vi "Dequeue Master and Local.vi"(8 "error in (no error)":errorcluster, 10 "Master Queue In":refnum<queue>, 11 "UI In":refnum<queue>) -> (0 "error out":errorcluster, 1 "Message Data":variant, 2 "Message":string, 3 "UI Out":refnum<queue>)   [LabVIEW 2013, in "Cal Inst.lvlib" / "Cal Inst Message Queue.lvlib"]
uses:
  Cal Inst Message Queue.lvlib
  Message Cluster.ctl
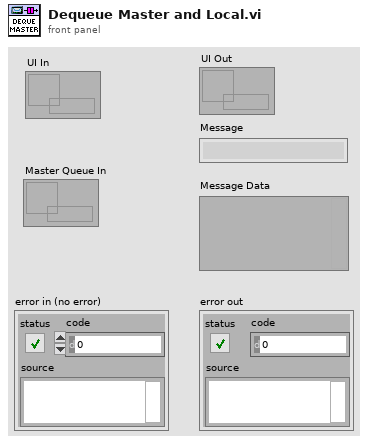
[diagram p1: front panel]
types:
  T1 = typedef "Cal Inst.lvlib/Cal Inst Message Queue.lvlib/Message Cluster.ctl" = cluster{"Message":string, "Message Data":variant}
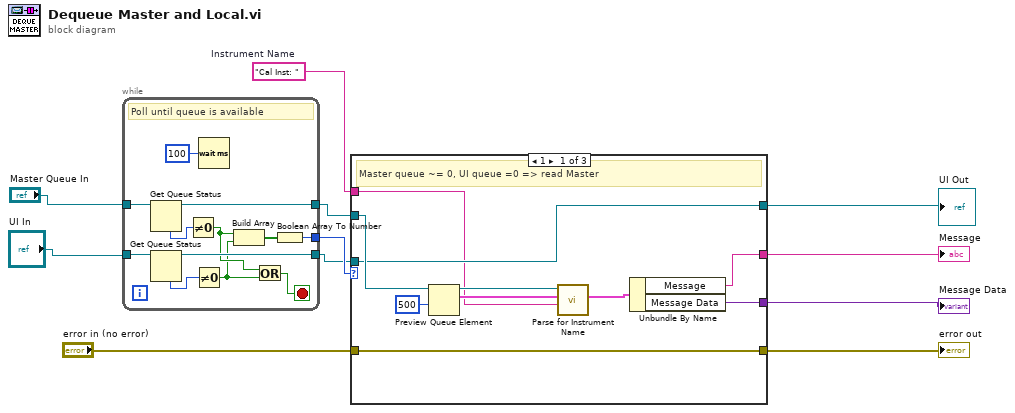
[diagram p0: block diagram]
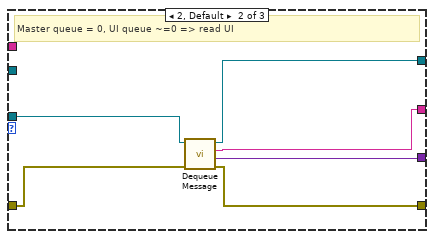
[diagram p2: hidden frame]
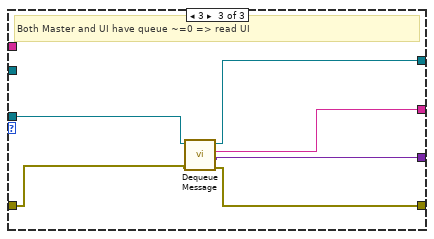
[diagram p3: hidden frame]
diagram:
  w6 = "Cal Inst: "  # Instrument Name
  n1 = while {
    tunnel: "UI In" -> [w23]
    tunnel: "Master Queue In" -> [w20]
    tunnel: [w18] -> w11
    tunnel: [w17] -> w10
    tunnel: [w16] -> w9
    stop <- w14 stop-if-true
    # "Poll until queue is available"
    n2 = Get Queue Status(queue=w20) -> (queue out=w17:refnum<queue>, # elements in queue=w21:i32)  [unwired: 2 in, 6 out]
    n3 = Get Queue Status(queue=w23) -> (queue out=w16:refnum<queue>, # elements in queue=w22:i32)  [unwired: 2 in, 6 out]
    n4 = Not Equal To 0?(x=w21) -> (x != 0?=w13:bool)
    n5 = Not Equal To 0?(x=w22) -> (x != 0?=w12:bool)
    n6 = Wait (ms)(milliseconds to wait=u32 100) -> ()  [unwired: 1 out]
    n7 = Build Array(w13, w12) -> (w19:bool[])
    n8 = Or(x=w13, y=w12) -> (x .or. y?=w14:bool)
    n9 = Boolean Array To Number(Boolean array=w19) -> (number=w18:u32)
  }
  n10 = case shown="1" w11 {
    tunnel: w10 -> [w30 _ _]
    tunnel: w9 -> [w26 w39 w40]
    tunnel: "error in (no error)" -> [w31 w38 w45]
    tunnel: [w26 w34 w41] -> w3
    tunnel: [w33 w35 w42] -> w2
    tunnel: [w32 w36 w43] -> w1
    tunnel: [w31 w37 w44] -> w7
    tunnel: w6 -> [w25 _ _]
    frame 1 {
      # "Master queue ~= 0, UI queue =0 => read Master"
      n11 = Preview Queue Element(queue=w30, timeout in ms (-1)=500) -> (queue out=w29:refnum<queue>, element=w28:T1)  [unwired: 1 in, 2 out]
      n12 = call "Parse for Instrument Name.vi"("Instrument Name"=w25, "Message In"=w28, "Message Queue"=w29) -> ("Message Out"=w27:T1)  [unwired: 8 in]
      n13 = Unbundle By Name(w27) -> ("Message"=w33:string, "Message Data"=w32:variant)
    }
    frame 2, Default {
      # "Master queue = 0, UI queue ~=0 => read UI"
      n14 = call "Dequeue Message.vi"("error in (no error)"=w38, "Message Queue"=w39) -> ("error out"=w37:errorcluster, "Message Data"=w36:variant, "Message"=w35:string, "dup Message Queue"=w34:refnum<queue>)  [unwired: 6 in]
    }
    frame 3 {
      # "Both Master and UI have queue ~=0 => read UI"
      n15 = call "Dequeue Message.vi"("error in (no error)"=w45, "Message Queue"=w40) -> ("error out"=w44:errorcluster, "Message Data"=w43:variant, "Message"=w42:string, "dup Message Queue"=w41:refnum<queue>)  [unwired: 6 in]
    }
  }
  "error out" <- w7
  "UI Out" <- w3
  "Message" <- w2
  "Message Data" <- w1
